vi "running average.vi"(5 "Initialize? (F)":bool, 7 "Averaging Size":i32, 9 "Average Type(FIR)":T1, 11 "Value":dbl) -> (3 "Average":dbl)   [LabVIEW 2011]
uses:
  <userlib>/_MGI/1D Array/MGI Average Type Enum.ctl
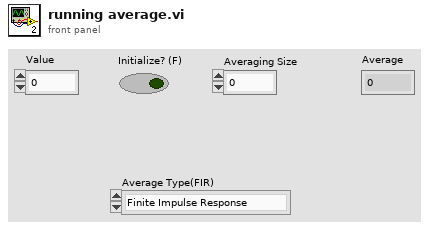
[diagram p1: front panel]
types:
  T1 = typedef "MGI Average Type Enum.ctl" = enum16{"Finite Impulse Response", "Infinite Impulse Response"}
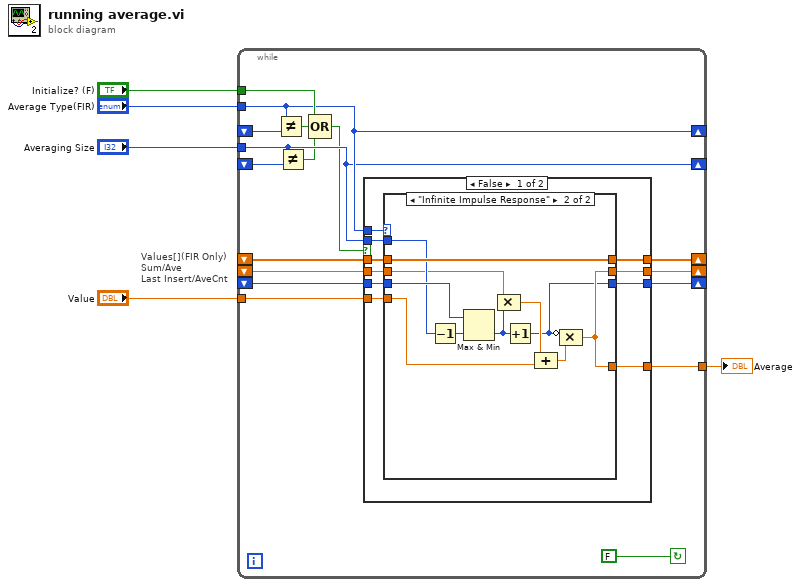
[diagram p0: block diagram]
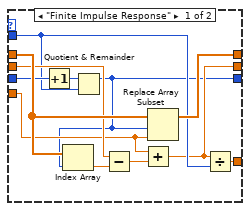
[diagram p2: hidden frame]
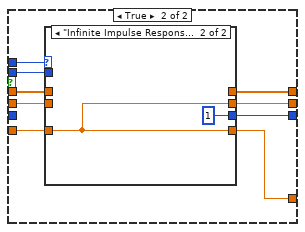
[diagram p3: hidden frame]
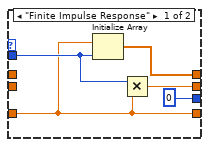
[diagram p4: hidden frame]
diagram:
  # "Values[](FIR Only)\nSum/Ave\nLast Insert/AveCnt"
  n1 = while {
    tunnel: "Averaging Size" -> [w9]
    tunnel: "Value" -> [w11]
    shift-left: _ -> [w15]
    shift-right: [w17] -> _
    tunnel: "Initialize? (F)" -> [w20]
    shift-left: _ -> [w14]
    shift-right: [w13] -> _
    tunnel: "Average Type(FIR)" -> [w10]
    shift-right: [w10] -> _
    shift-left: _ -> [w21]
    shift-right: [w18] -> _
    shift-left: _ -> [w16]
    shift-right: [w9] -> _
    shift-left: _ -> [w19]
    tunnel: [w12] -> w2
    stop <- FALSE continue-if-true
    n2 = Not Equal?(x=w10, y=w21) -> (x != y?=w8:bool)
    n3 = Not Equal?(x=w9, y=w19) -> (x != y?=w6:bool)
    n4 = Compound Arithmetic op=OR(w20, w8, w6) -> (w7:bool)
    n5 = case shown="False" w7 {
      tunnel: [w26 w56] -> w18
      tunnel: w11 -> [w28 w59]
      tunnel: [w24 w58] -> w17
      tunnel: w16 -> [w31 _]
      tunnel: w15 -> [w30 w62]
      tunnel: w14 -> [w29 w60]
      tunnel: w9 -> [w27 w63]
      tunnel: w10 -> [w32 w64]
      tunnel: [w25 w61] -> w13
      tunnel: [w23 w57] -> w12
      frame False {
        n6 = case shown="\"Infinite Impulse Response\"" w32 {
          tunnel: w31 -> [w42 w54]
          tunnel: w30 -> [w41 w51]
          tunnel: w29 -> [w43 w55]
          tunnel: w28 -> [w37 w50]
          tunnel: w27 -> [w36 w53]
          tunnel: [w33 w45] -> w26
          tunnel: [w39 w55] -> w25
          tunnel: [w35 w47] -> w24
          tunnel: [w34 w47] -> w23
          frame "Finite Impulse Response" {
            n7 = Increment(x=w42) -> (x+1=w44:i32)
            n8 = Quotient & Remainder(x=w44, y=w36) -> (x-y*floor(x/y)=w33:i32)  [unwired: 1 out]
            n9 = Index Array(array=w43, index=w33) -> (element=w40:dbl)
            n10 = Subtract(x=w41, y=w40) -> (x-y=w38:dbl)
            n11 = Add(x=w37, y=w38) -> (x+y=w35:dbl)
            n12 = Replace Array Subset(array=w43, new element=w37, index=w33) -> (w39:dbl[])
            n13 = Divide(x=w35, y=w36) -> (x/y=w34:dbl)
          }
          frame "Infinite Impulse Response" {
            n14 = Decrement(x=w53) -> (x-1=w52:i32)
            n15 = Max & Min(x=w54, y=w52) -> (min(x,y)=w46:i32)  [unwired: 1 out]
            n16 = Compound Arithmetic op=MULTIPLY(w51, w46) -> (w49:dbl)
            n17 = Increment(x=w46) -> (x+1=w45:i32)
            n18 = Compound Arithmetic op=ADD(w49, w50) -> (w48:dbl)
            n19 = Compound Arithmetic op=MULTIPLY(invert w45, w48) -> (w47:dbl)
          }
        }
      }
      frame True {
        n20 = case shown="\"Infinite Impulse Response\"" w64 {
          tunnel: w63 -> [w68 _]
          tunnel: w62 -> [_ _]
          tunnel: [w69 _] -> w61
          tunnel: w60 -> [_ _]
          tunnel: w59 -> [w66 w71]
          tunnel: [w67 w71] -> w58
          tunnel: [w66 w71] -> w57
          tunnel: [0 1] -> w56
          frame "Finite Impulse Response" {
            n21 = Initialize Array(w66, w68) -> (w69:dbl[])
            n22 = Multiply(x=w68, y=w66) -> (x*y=w67:dbl)
          }
          frame "Infinite Impulse Response" {
          }
        }
      }
    }
  }
  "Average" <- w2
